vi "DashboardCore.vi"(8 "Robot IP notifier in":refnum<notifier>, 9 "Window mode notifier in":refnum<notifier>, 11 "Main Dashboard tab":refnum<vi>) -> ()   [LabVIEW 2015]
panel:
  in  "TCP":refnum<k5>
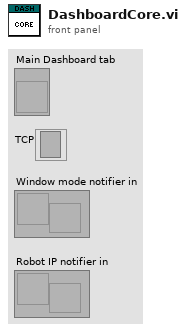
[diagram p1: front panel]
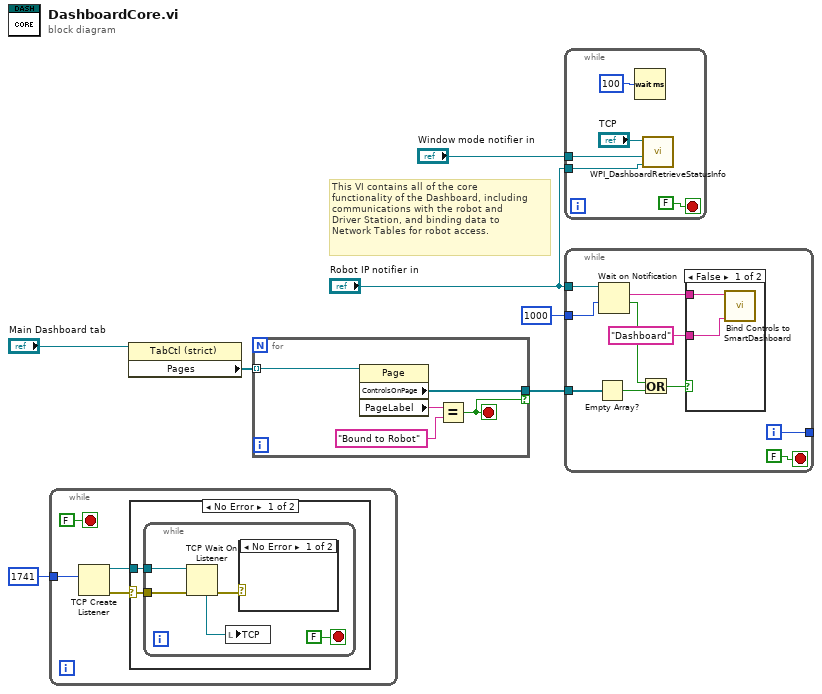
[diagram p0: block diagram]
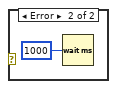
[diagram p2: hidden frame]
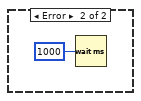
[diagram p3: hidden frame]
diagram:
  # "This VI contains all of the core\nfunctionality of the Dashboard, including\ncommunications with the robot and\nDriver Station, and binding data to \nNetwork Tables for robot access."
  n1 = while {
    tunnel: u16 1741 ("timeout ms (25000)") -> [w9]
    stop <- FALSE stop-if-true
    n2 = TCP Create Listener(10:w9) -> (0:w8:errorcluster, 3:w10:refnum<k5>)  [unwired: 4 in, 1 out]
    n3 = case shown="No Error" w8 {
      selector: w8 -> [w12 _]
      tunnel: w10 -> [w13 _]
      frame No Error {
        n4 = while {
          tunnel: w13 -> [w17]
          tunnel: w12 -> [w16]
          stop <- FALSE stop-if-true
          n5 = TCP Wait On Listener(8:w16, 11:w17) -> (0:w18:errorcluster, 4:w14:refnum<k5>)  [unwired: 2 in, 3 out]
          n6 = local write "TCP"(w14) -> ()
          n7 = case shown="No Error" w18 {
            frame No Error {
            }
            frame Error {
              n8 = Wait (ms)(milliseconds to wait=u32 1000) -> ()  [unwired: 1 out]
            }
          }
        }
      }
      frame Error {
        n9 = Wait (ms)(milliseconds to wait=u32 1000) -> ()  [unwired: 1 out]
      }
    }
  }
  n10 = property on="Property Node" class="TabCtl (strict)"(reference="Main Dashboard tab") -> ("Pages"=w2:refnum<vi>[])  [unwired: 1 in, 2 out]
  n11 = for {
    tunnel: w2 -> [w25] mode=indexing
    tunnel: [w22] -> w1 if=w21
    stop <- w21 stop-if-true
    n12 = property class="Page"(reference=w25) -> ("ControlsOnPage"=w22:refnum<vi>[], "PageLabel"=w24:string)  [unwired: 1 in, 2 out]
    n13 = Equal?(x=w24, y="Bound to Robot" ("element")) -> (x = y?=w21:bool)
  }
  n14 = while {
    tunnel: "Window mode notifier in" -> [w29]
    tunnel: "Robot IP notifier in" -> [w28]
    stop <- FALSE stop-if-true
    n15 = Wait (ms)(milliseconds to wait=u32 100) -> ()  [unwired: 1 out]
    n16 = call <vilib>:"WPI_DashboardRetrieveStatusInfo.vi"("Binding Refnum"=w28, "Window Mode Notifier"=w29, "TCP Cnx"="TCP") -> ()  [unwired: 3 in, 6 out]
  }
  n17 = while {
    tunnel: "Robot IP notifier in" -> [w39]
    tunnel: [w37] -> _
    tunnel: u32 1000 ("milliseconds to wait") -> [w36]
    tunnel: w1 -> [w31]
    i -> [w37]
    stop <- FALSE stop-if-true
    n18 = Empty Array?(array=w31) -> (empty?=w33:bool)
    n19 = Wait on Notification(notifier=w39, timeout in ms (-1)=w36) -> (notification=w38:string, timed out?=w32:bool)  [unwired: 2 in, 2 out]
    n20 = Or(x=w32, y=w33) -> (x .or. y?=w34:bool)
    n21 = case shown="False" w34 {
      tunnel: w38 -> [w42 _]
      tunnel: "Dashboard" -> [w41 _]
      frame False {
        n22 = call <vilib>:"Bind Controls to SmartDashboard.vi"("Client Name"=w41, "Server IP Address"=w42) -> ()  [unwired: 10 in]
      }
      frame True {
      }
    }
  }
